vi "[SubV]Gait_Phase_Estimate_R.vi"(2 "Index":i32, 3 "Hill Contact":bool) -> (0 "GP":dbl, 1 "Cadence":dbl)   [LabVIEW 2019]
uses:
  <vilib>/Analysis/baseanly.llb/Mean (DBL).vi
  <vilib>/Analysis/NI_AALBase.lvlib
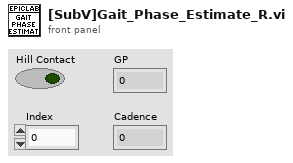
[diagram p1: front panel]
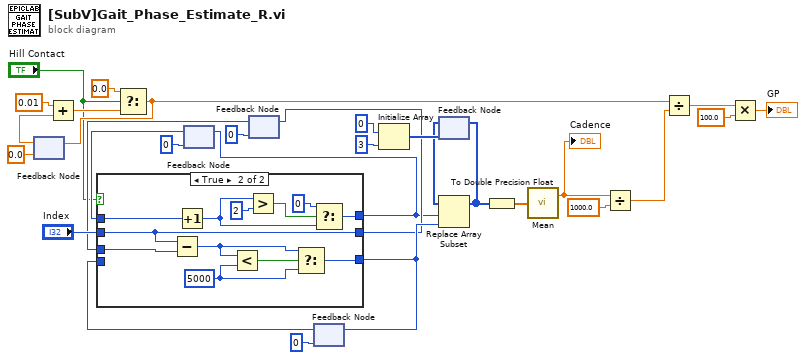
[diagram p0: block diagram]
diagram:
  n1 = feedback #1(0.0 ("t")) -> (w7:dbl)
  n2 = Add(x=0.01, y=w7) -> (x+y=w8:dbl)
  n3 = Select(t=0.0, s="Hill Contact", f=w8) -> (s? t:f=w5:dbl)
  n4 = feedback-in #1(w5) -> ()
  n5 = feedback #2(0 ("t")) -> (w11:i32)
  n6 = feedback #3(0 ("Index")) -> (w12:i32)
  n7 = feedback #4(0 ("y")) -> (w18:i32)
  n8 = case shown="True" "Hill Contact" {
    tunnel: w11 -> [w32 w42]
    tunnel: [w32 w41] -> w10
    tunnel: w12 -> [w31 w36]
    tunnel: "Index" -> [_ w37]
    tunnel: [w31 w37] -> w13
    tunnel: [w30 w35] -> w24
    tunnel: w18 -> [w30 _]
    frame False {
    }
    frame True {
      w33 = 5000 ("y")
      n9 = Subtract(x=w37, y=w36) -> (x-y=w34:i32)
      n10 = Increment(x=w42) -> (x+1=w40:i32)
      n11 = Less?(x=w34, y=w33) -> (x < y?=w38:bool)
      n12 = Greater?(x=w40, y=2) -> (0:w44:bool)
      n13 = Select(t=w34, s=w38, f=w33) -> (s? t:f=w35:i32)
      n14 = Select(t=0, s=w44, f=w40) -> (s? t:f=w41:i32)
    }
  }
  n15 = feedback-in #2(w10) -> ()
  n16 = feedback-in #3(w13) -> ()
  n17 = feedback-in #4(w24) -> ()
  n18 = Initialize Array(0 ("dimension size"), 3 ("dimension size")) -> (w21:i32[])
  n19 = feedback #5(w21) -> (w14:i32[])
  n20 = Replace Array Subset(array=w14, new element=w24, index=w10) -> (w15:i32[])
  n21 = feedback-in #5(w15) -> ()
  n22 = To Double Precision Float(number=w15) -> (double precision float=w16:dbl[])
  n23 = call-poly <vilib>:"Mean.vi"("X"=w16) -> ("mean"=w22:dbl)  [unwired: 1 out]
  "Cadence" <- w22
  n24 = Divide(x=w22, y=1000.0) -> (x/y=w26:dbl)
  n25 = Divide(x=w5, y=w26) -> (x/y=w25:dbl)
  n26 = Multiply(x=w25, y=100.0) -> (x*y=→"GP":dbl)
